vi "Linea idraulica selezionata.vi"() -> ()   [LabVIEW 2019]
panel:
  out "Banco":i32
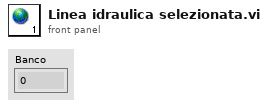
[diagram p1: front panel]
diagram:
